vi "TDTRX6-Init DAQ.vi"(0 "AO Fs (Hz)":dbl, 5 "AI Fs (Hz)":dbl, 7 "T (ms)":dbl, 9 "Num AO Buffers":i32=2, 11 "error in (no error)":errorcluster, 12 "AI Channels":i32[](array[numeric])=[1, 2]) -> (4 "AO Fs (coerced)":dbl, 6 "AI Fs (coerced)":dbl, 8 "AO npts":i32, 10 "AI npts":i32, 15 "error out":errorcluster)   [LabVIEW 2020]
uses:
  TDT-Signal Bank Action.ctl
  TDT-Globals.vi
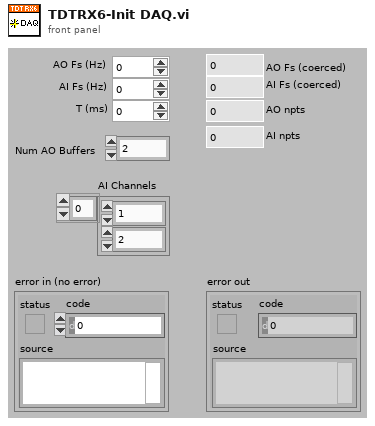
[diagram p1: front panel]
types:
  T1 = typedef "TDT-Signal Bank Action.ctl" = enum16{"Init", "Write", "Read", "Rewrite", "Reset", "Recycle", "Ramp up", "Ramp down", "Zero"}
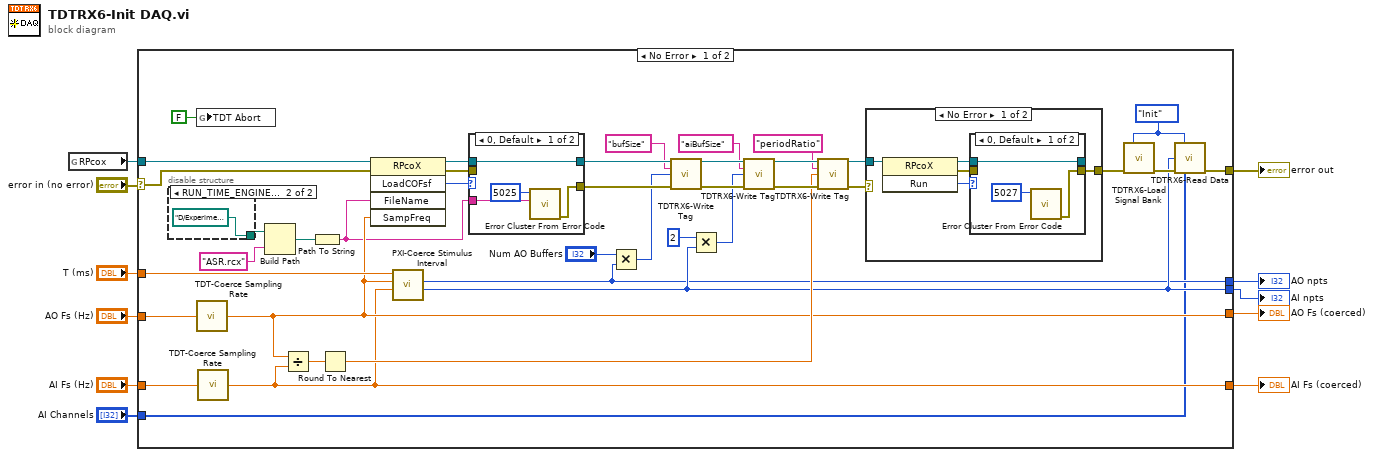
[diagram p0: block diagram]
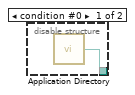
[diagram p2: hidden frame]
diagram:
  n1 = global read "TDT-Globals.vi" "RPcox"() -> (w1:refnum<k7>)
  n2 = case shown="No Error" "error in (no error)" {
    selector: "error in (no error)" -> [w48 w70]
    tunnel: [w23 w70] -> w10
    tunnel: w1 -> [w13 _]
    tunnel: "AO Fs (Hz)" -> [w29 _]
    tunnel: "AI Fs (Hz)" -> [w28 _]
    tunnel: "T (ms)" -> [w26 _]
    tunnel: [w25 _] -> w6
    tunnel: [w24 _] -> w5
    tunnel: [w17 _] -> w4
    tunnel: [w20 _] -> w3
    tunnel: "AI Channels" -> [w14 _]
    frame No Error {
      w22 = TDT-Signal_Bank_Action."Init" ("Action")
      n3 = disable-structure shown="RUN_TIME_ENGINE==False" {
        disable-tunnel: [w51 path "D:/Experiment VIs/PXI DAQ VIs/TDT VIs/rpfiles"] -> w12
        frame condition #0 {
          n4 = call <vilib>:"Application Directory.vi"() -> ("Application Directory"=w51:path)
        }
        frame condition #1 (active) {
        }
      }
      n5 = global write "TDT-Globals.vi" "TDT Abort"(FALSE ("TDT Abort")) -> ()
      n6 = call "TDT-Coerce Sampling Rate.vi"("Fs (Hz)"=w29) -> ("Coerced"=w25:dbl)
      n7 = call "TDT-Coerce Sampling Rate.vi"("Fs (Hz)"=w28) -> ("Coerced"=w24:dbl)
      n8 = Build Path(base path=w12, name or relative path="ASR.rcx") -> (appended path=w49:path)
      n9 = Divide(x=w25, y=w24) -> (x/y=w30:dbl)
      n10 = Path To String(path=w49) -> (string=w15:string)
      n11 = Round To Nearest(number=w30) -> (nearest integer value=w27:dbl)
      n12 = invoke class="RPcoX" method="LoadCOFsf"(reference=w13, error in=w48, "FileName"=w15, "SampFreq"=w25) -> (reference out=w46:refnum<k7>, error out=w45:errorcluster, "LoadCOFsf"=w47:i32)  [unwired: 1 in, 2 out]
      n13 = call "PXI-Coerce Stimulus Interval.vi"("AI sampling rate (Hz)"=w24, "AO sampling rate (Hz)"=w25, "Stimulus interval (ms)"=w26) -> ("AI npts"=w20:i32, "AO npts"=w17:i32)  [unwired: 5 in, 2 out]
      n14 = case shown="0, Default" w47 {
        tunnel: w15 -> [w66 _]
        tunnel: w46 -> [w67 w69]
        tunnel: w45 -> [_ w68]
        tunnel: [w67 w69] -> w44
        tunnel: [w64 w68] -> w43
        frame 0, Default {
          n15 = call <vilib>:"Error Cluster From Error Code.vi"("error message (\"\")"=w66, "error code (0)"=5025) -> ("error out"=w64:errorcluster)  [unwired: 7 in]
        }
        frame 1 {
        }
      }
      n16 = Multiply(x="Num AO Buffers", y=w17) -> (x*y=w18:i32)
      n17 = call "TDTRX6-Write Tag.vi"("RPcox"=w44, "Name"="bufSize", "Value"=w18, "error in"=w43) -> ("RPcox Out"=w40:refnum<k7>, "error out"=w41:errorcluster)  [unwired: 10 in]
      n18 = Multiply(x=2, y=w20) -> (x*y=w21:i32)
      n19 = call "TDTRX6-Write Tag.vi"("RPcox"=w40, "Name"="aiBufSize", "Value"=w21, "error in"=w41) -> ("RPcox Out"=w37:refnum<k7>, "error out"=w38:errorcluster)  [unwired: 10 in]
      n20 = call "TDTRX6-Write Tag.vi"("RPcox"=w37, "Name"="periodRatio", "Value"=w27, "error in"=w38) -> ("RPcox Out"=w35:refnum<k7>, "error out"=w33:errorcluster)  [unwired: 10 in]
      n21 = case shown="No Error" w33 {
        selector: w33 -> [_ w63]
        tunnel: w35 -> [w57 _]
        tunnel: [w54 w63] -> w34
        frame No Error {
          n22 = invoke class="RPcoX" method="Run"(reference=w57) -> (reference out=w55:refnum<k7>, error out=w56:errorcluster, "Run"=w53:i32)  [unwired: 2 in]
          n23 = case shown="0, Default" w53 {
            tunnel: w55 -> [w60 w62]
            tunnel: w56 -> [_ w61]
            tunnel: [w60 w62] -> _
            tunnel: [w58 w61] -> w54
            frame 0, Default {
              n24 = call <vilib>:"Error Cluster From Error Code.vi"("error code (0)"=5027) -> ("error out"=w58:errorcluster)  [unwired: 8 in]
            }
            frame 1 {
            }
          }
        }
        frame Error {
        }
      }
      n25 = call "TDTRX6-Load Signal Bank.vi"("Action"=w22, "error in (no error)"=w34) -> ("error out"=w32:errorcluster)  [unwired: 13 in]
      n26 = call "TDTRX6-Read Data.vi"("Action"=w22, "Pts Per Read"=w20, "error in (no error)"=w32, "AI Channels"=w14) -> ("error out"=w23:errorcluster)  [unwired: 10 in, 1 out]
    }
    frame Error {
    }
  }
  "error out" <- w10
  "AO Fs (coerced)" <- w6
  "AI Fs (coerced)" <- w5
  "AO npts" <- w4
  "AI npts" <- w3
